vi "getRPM.vi"() -> ()   [LabVIEW 2019]
panel:
  out "Waveform Graph":dynamicdata(graph)
  out "Numeric":dbl
  in  "stop (F)":bool
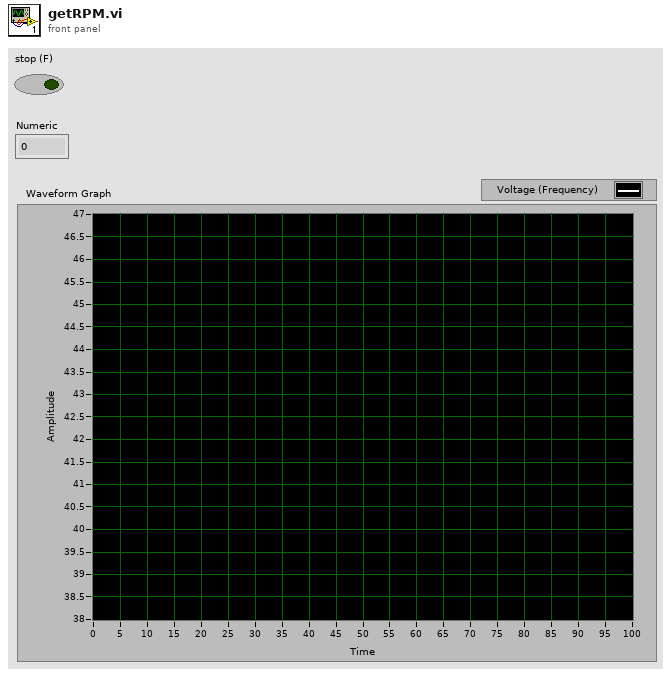
[diagram p1: front panel]
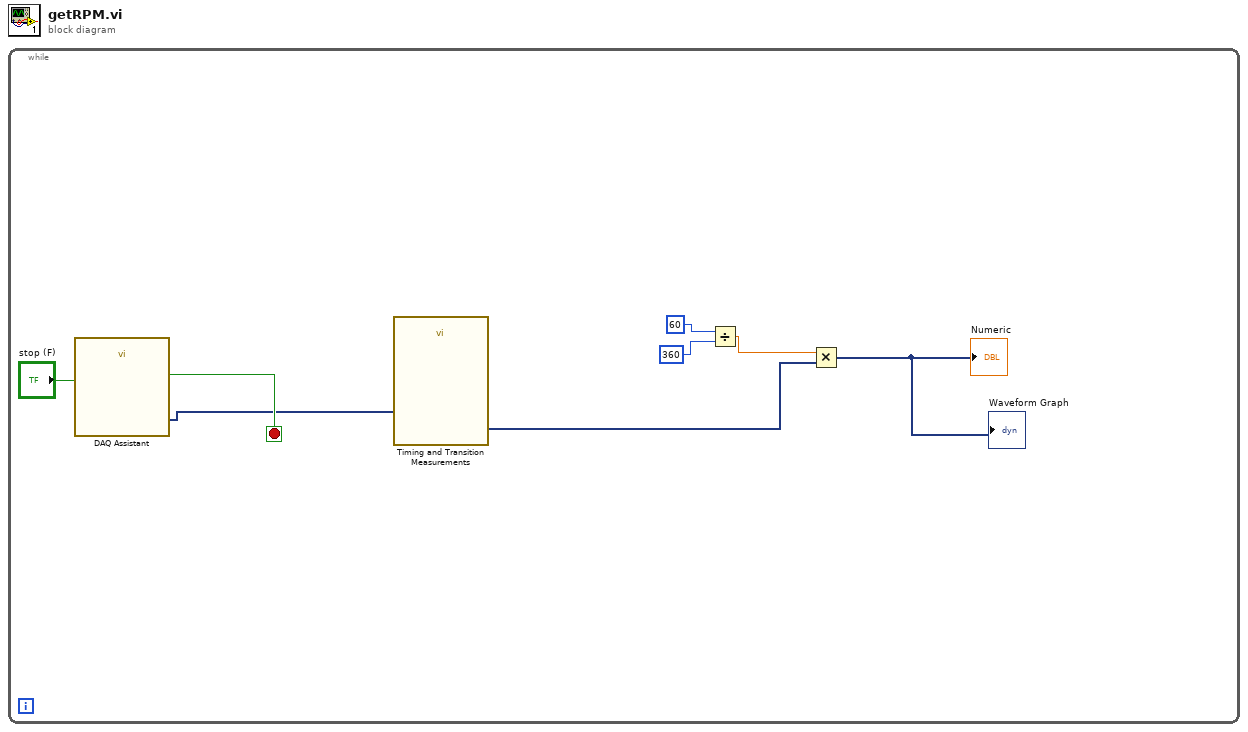
[diagram p0: block diagram]
diagram:
  n1 = while {
    stop <- w7 stop-if-true
    n2 = call "DAQ Assistant"("stop (F)"="stop (F)") -> ("data"=w6:dynamicdata, "stopped"=w7:bool)  [unwired: 15 in, 2 out]
    n3 = call "Timing and Transition Measurements"("Signals"=w6) -> ("Frequency"=w4:dynamicdata)  [unwired: 9 in, 1 out]
    n4 = Divide(x=60, y=360) -> (x/y=w5:dbl)
    n5 = Multiply(x=w5, y=w4) -> (x*y=→"Numeric" →"Waveform Graph":dynamicdata)
  }
